vi "Remove and Rewire Objects_core.vi"(8 "error in (no error)":errorcluster, 10 "Clean Wires (T)":bool=TRUE, 11 "Items to Remove":refnum<vi>[](array[refnum])) -> (0 "error out":errorcluster, 3 "Any Items Removed?":bool)   [LabVIEW 2020]
uses:
  <vilib>/Utility/Data Type/Type Definitions/Data Type.ctl
  <vilib>/Utility/Data Type/NI_Data Type.lvlib
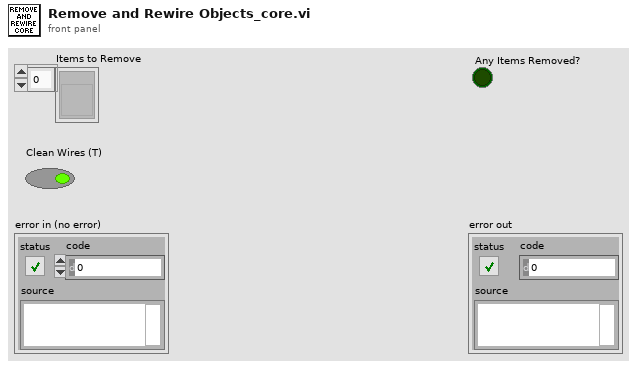
[diagram p1: front panel]
types:
  T1 = typedef "NI_Data Type.lvlib/Data Type.ctl" = enum8{"Invalid Type", "Void", "I8", "I16", "I32", "I64", "U8", "U16", "U32", "U64", "Single Float", "Double Float", "Extended Float", "Single Complex", "Double Complex", "Extended Complex", "Enum U8", "Enum U16", "Enum U32", "Enum U64", "Single Float With Unit", "Double Float With Unit", "Extended Float With Unit", "Single Complex with Unit", "Double Complex with Unit", "Extended Complex with Unit", "Boolean", "String", "Path", "Picture", "Tag", "Array", "Cluster", "Variant", "LV Variant", "Waveform", "Timestamp", "Digital Waveform", "Digital Data", "ExpressData", "Refnum", "External Data", "VI", "Poly VI", "LabVIEW Class Instance", "Fixed Point", "Set Collection", "Map Collection"}
  T2 = cluster{"Left":i32, "Top":i32, "Terminal":refnum<vi>}
  T3 = cluster{"Left":i32, "Top":i32, "Terminal":refnum<vi>}[]
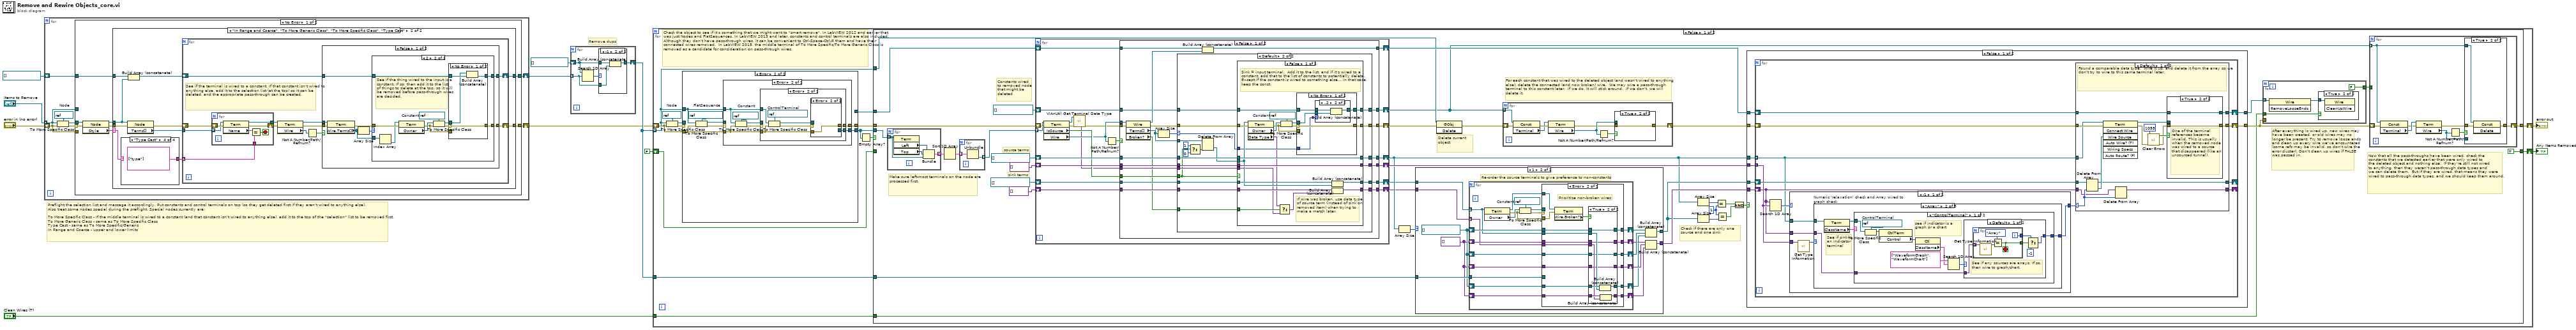
[diagram p0: block diagram]
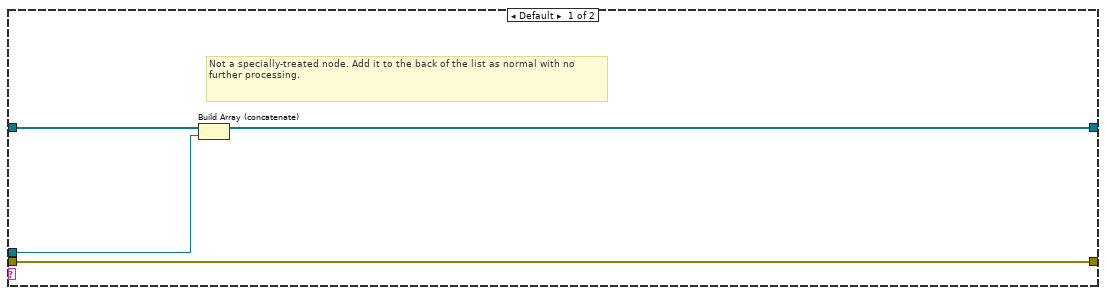
[diagram p3: hidden frame]
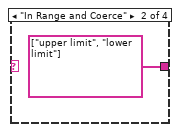
[diagram p5: hidden frame]
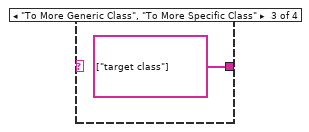
[diagram p6: hidden frame]
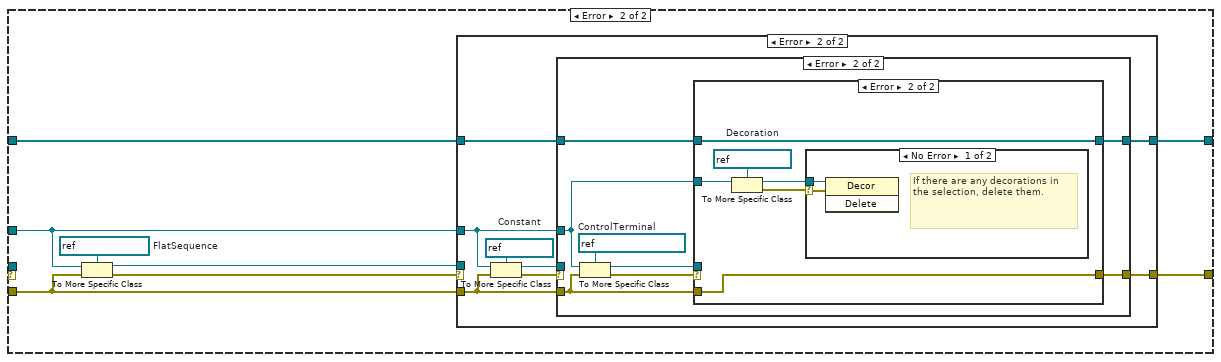
[diagram p10: hidden frame]
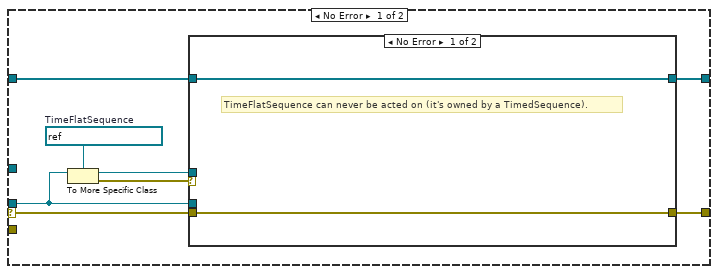
[diagram p11: hidden frame]
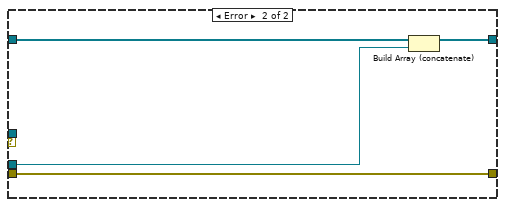
[diagram p12: hidden frame]
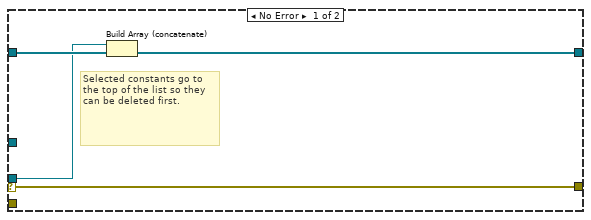
[diagram p13: hidden frame]
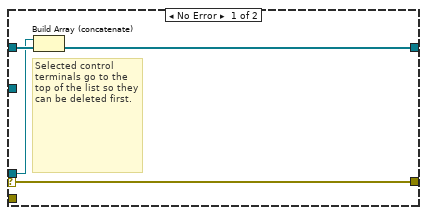
[diagram p14: hidden frame]
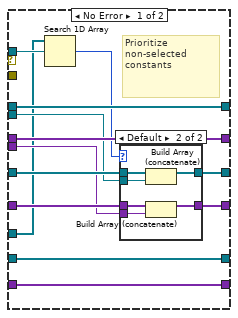
[diagram p17: hidden frame]
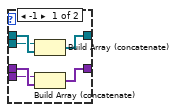
[diagram p18: hidden frame]
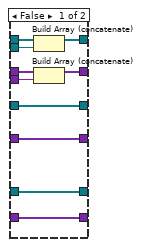
[diagram p19: hidden frame]
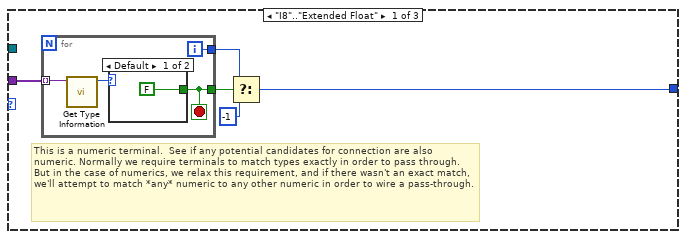
[diagram p20: hidden frame]
diagram:
  # "Preflight the selection list and massage it accordingly. Put constants and control terminals on top (so they get deleted first if they aren't wired to anything else).\nAlso treat some nodes special during the preflight. Special nodes currently are:\n\nTo More Specific Class - If the middle terminal is wired to a constant (and that constant isn't wired to anything else), add it to the top of the \"selection\" list to be removed first.\nTo More Generic Class - same as To More Specific Class\nType Cast - same as To More Specific/Generic\nIn Range and Coerce - upper and lower limits"
  # "Remove dups"
  n1 = for {
    tunnel: "Items to Remove" -> [w13] mode=indexing
    shift-right: [w14] -> w7
    shift-left: "error in (no error)" -> [w17]
    shift-right: [w15] -> w9
    shift-left: refnum<vi>[] [] ("SelList[]") -> [w16]
    w12 = refnum<vi> refnum  # Node
    n2 = To More Specific Class(target class=w12, reference=w13, error in=w17) -> (specific class reference=w19:refnum<vi>, error out=w18:errorcluster)
    n3 = case shown="No Error" w18 {
      selector: w18 -> [w27 _]
      tunnel: w19 -> [w26 _]
      tunnel: [w20 w98] -> w14
      tunnel: w13 -> [_ w96]
      tunnel: w17 -> [_ w97]
      tunnel: w16 -> [w22 w95]
      tunnel: [w21 w94] -> w15
      frame No Error {
        n4 = property class="Node"(reference=w26, error in=w27) -> (reference out=w23:refnum<vi>, error out=w24:errorcluster, "Style"=w25:string)
        n5 = case shown="\"In Range and Coerce\", \"To More Generic Class\", \"To More Specific Class\", \"Type Cast\"" w25 {
          selector: w25 -> [_ w32]
          tunnel: w24 -> [w29 w40]
          tunnel: w23 -> [w28 w39]
          tunnel: w22 -> [w31 w41]
          tunnel: [w30 w35] -> w21
          tunnel: [w29 w34] -> w20
          frame Default {
            # "Not a specially-treated node. Add it to the back of the list as normal with no further processing."
            n6 = Build Array (concatenate)(w31, w28) -> (w30:refnum<vi>[])
          }
          frame "In Range and Coerce", "To More Generic Class", "To More Specific Class", "Type Cast" {
            n7 = case shown="\"Type Cast\"" w32 {
              tunnel: [_ string[] ["upper limit", "lower limit"] string[] ["target class"] string[] ["type"]] -> w33
              frame Default {
              }
              frame "In Range and Coerce" {
              }
              frame "To More Generic Class", "To More Specific Class" {
              }
              frame "Type Cast" {
              }
            }
            n8 = property class="Node"(reference=w39, error in=w40) -> (error out=w38:errorcluster, "Terms[]"=w37:refnum<vi>[])  [unwired: 1 out]
            n9 = Build Array (concatenate)(w41, w39) -> (w36:refnum<vi>[])
            n10 = for {
              tunnel: w37 -> [w55]
              shift-right: [w51] -> w34
              shift-left: w38 -> [w56]
              shift-right: [w52] -> w35
              shift-left: w36 -> [w53]
              tunnel: w33 -> [w45] mode=indexing
              # "See if the terminal is wired to a constant. If that constant isn't wired to anything else, add it to the selection list (at the top) so it can be deleted, and the appropriate pass-through can be created."
              n11 = for {
                tunnel: w55 -> [w91] mode=indexing
                tunnel: [w89] -> w49
                shift-right: [w88] -> w54
                shift-left: w56 -> [w92]
                tunnel: w45 -> [w86]
                stop <- w87 stop-if-true
                n12 = property class="Term"(reference=w91, error in=w92) -> (reference out=w89:refnum<vi>, error out=w88:errorcluster, "Name"=w90:string)
                n13 = Equal?(x=w90, y=w86) -> (x = y?=w87:bool)
              }
              n14 = property class="Term"(reference=w49, error in=w54) -> (reference out=w48:refnum<vi>, error out=w50:errorcluster, "Wire"=w47:refnum<vi>)
              n15 = Not A Number/Path/Refnum?(number/path/refnum=w47) -> (NaN/Path/Refnum?=w46:bool)
              n16 = case shown="False" w46 {
                tunnel: w53 -> [w64 w85]
                tunnel: [w61 w85] -> w52
                tunnel: [w60 w84] -> w51
                tunnel: w50 -> [w58 w84]
                tunnel: w48 -> [w57 _]
                frame False {
                  n17 = property class="Term"(reference=w57, error in=w58) -> (error out=w63:errorcluster, "Wire.Terms[]"=w59:refnum<vi>[])  [unwired: 1 out]
                  n18 = Array Size(array=w59) -> (size(s)=w62:i32)
                  n19 = case shown="2" w62 {
                    tunnel: w64 -> [w66 w71]
                    tunnel: w63 -> [w65 w76]
                    tunnel: [w66 w70] -> w61
                    tunnel: [w65 w68] -> w60
                    tunnel: w59 -> [_ w77]
                    frame Default {
                      # "Any number of terminals on the upper/lower limit wires other than 2 means that whatever is wired to it, is also wired to something else. Don't try to delete that thing in this case."
                    }
                    frame 2 {
                      w73 = refnum<vi> refnum  # Constant
                      # "See if the thing wired to the input is a constant. If so, then add it to the list of things to delete at the top, so it will be removed before pass-through wires are decided."
                      n20 = Index Array(array=w77) -> (element=w75:refnum<vi>)  [unwired: 1 in]
                      n21 = property class="Term"(reference=w75, error in=w76) -> (error out=w69:errorcluster, "Owner"=w74:refnum<vi>)  [unwired: 1 out]
                      n22 = To More Specific Class(target class=w73, reference=w74, error in=w69) -> (specific class reference=w67:refnum<vi>, error out=w72:errorcluster)
                      n23 = case shown="No Error" w72 {
                        selector: w72 -> [w79 _]
                        tunnel: w71 -> [w81 w83]
                        tunnel: [w80 w83] -> w70
                        tunnel: w69 -> [_ w82]
                        tunnel: [w79 w82] -> w68
                        tunnel: w67 -> [w78 _]
                        frame No Error {
                          n24 = Build Array (concatenate)(w78, w81) -> (w80:refnum<vi>[])
                        }
                        frame Error {
                        }
                      }
                    }
                  }
                }
                frame True {
                  # "Terminal is not wired...no further work necessary"
                }
              }
            }
          }
        }
      }
      frame Error {
        w93 = refnum<vi> refnum  # FlatSequence
        n25 = To More Specific Class(target class=w93, reference=w96, error in=w97) -> (specific class reference=w99:refnum<vi>, error out=w100:errorcluster)
        n26 = case shown="Error" w100 {
          selector: w100 -> [w103 _]
          tunnel: w99 -> [w105 _]
          tunnel: [w102 w118] -> w98
          tunnel: w97 -> [_ w119]
          tunnel: w96 -> [_ w120]
          tunnel: w95 -> [w108 w117]
          tunnel: [w107 w116] -> w94
          frame No Error {
            w106 = refnum<vi> refnum  # TimeFlatSequence
            n27 = To More Specific Class(target class=w106, reference=w105) -> (specific class reference=w101:refnum<vi>, error out=w104:errorcluster)  [unwired: 1 in]
            n28 = case shown="No Error" w104 {
              tunnel: w108 -> [w109 w114]
              tunnel: [w109 w113] -> w107
              tunnel: w105 -> [_ w112]
              tunnel: w103 -> [w110 w111]
              tunnel: [w110 w111] -> w102
              tunnel: w101 -> [_ _]
              frame No Error {
                # "TimeFlatSequence can never be acted on (it's owned by a TimedSequence)."
              }
              frame Error {
                n29 = Build Array (concatenate)(w114, w112) -> (w113:refnum<vi>[])
              }
            }
          }
          frame Error {
            w115 = refnum<vi> refnum  # Constant
            n30 = To More Specific Class(target class=w115, reference=w120, error in=w119) -> (specific class reference=w121:refnum<vi>, error out=w122:errorcluster)
            n31 = case shown="Error" w122 {
              selector: w122 -> [w126 _]
              tunnel: w121 -> [w123 _]
              tunnel: w120 -> [_ w127]
              tunnel: w119 -> [_ w132]
              tunnel: [w126 w131] -> w118
              tunnel: w117 -> [w125 w130]
              tunnel: [w124 w129] -> w116
              frame No Error {
                # "Selected constants go to the top of the list so they can be deleted first."
                n32 = Build Array (concatenate)(w123, w125) -> (w124:refnum<vi>[])
              }
              frame Error {
                w128 = refnum<vi> refnum  # ControlTerminal
                n33 = To More Specific Class(target class=w128, reference=w127, error in=w132) -> (specific class reference=w133:refnum<vi>, error out=w134:errorcluster)
                n34 = case shown="Error" w134 {
                  selector: w134 -> [w138 _]
                  tunnel: w133 -> [w135 _]
                  tunnel: w132 -> [_ w144]
                  tunnel: [w138 w144] -> w131
                  tunnel: w130 -> [w137 w143]
                  tunnel: [w136 w143] -> w129
                  tunnel: w127 -> [_ w142]
                  frame No Error {
                    # "Selected control terminals go to the top of the list so they can be deleted first."
                    n35 = Build Array (concatenate)(w135, w137) -> (w136:refnum<vi>[])
                  }
                  frame Error {
                    w141 = refnum<vi> refnum  # Decoration
                    n36 = To More Specific Class(target class=w141, reference=w142) -> (specific class reference=w139:refnum<vi>, error out=w140:errorcluster)  [unwired: 1 in]
                    n37 = case shown="No Error" w140 {
                      selector: w140 -> [w145 _]
                      tunnel: w139 -> [w146 _]
                      frame No Error {
                        # "If there are any decorations in the selection, delete them."
                        n38 = invoke class="Decor" method="Delete"(reference=w146, error in=w145) -> ()  [unwired: 1 in, 3 out]
                      }
                      frame Error {
                      }
                    }
                  }
                }
              }
            }
          }
        }
      }
    }
  }
  n39 = for {
    tunnel: w9 -> [w147] mode=indexing
    shift-right: [w148] -> w11
    shift-left: refnum<vi>[] [] ("SelList[]") -> [w149]
    n40 = Search 1D Array(1D array=w149, element=w147) -> (index of element=w150:i32)  [unwired: 1 in]
    n41 = case shown="-1" w150 {
      tunnel: w149 -> [w151 w154]
      tunnel: [w151 w153] -> w148
      tunnel: w147 -> [_ w152]
      frame Default {
      }
      frame -1 {
        n42 = Build Array (concatenate)(w154, w152) -> (w153:refnum<vi>[])
      }
    }
  }
  n43 = for {
    tunnel: w11 -> [w162] mode=indexing
    shift-right: [w161] -> w3
    shift-left: FALSE -> [w156]
    shift-right: [w160] -> w4
    shift-left: w7 -> [w166]
    tunnel: w11 -> [w159]
    tunnel: "Clean Wires (T)" -> [w155]
    w158 = refnum<vi> refnum  # Node
    # "Check the object to see if it's something that we might want to \"smart remove\". In LabVIEW 2012 and earlier that was just Nodes and FlatSequences. In LabVIEW 2013 and later, constants and control terminals are also included. Although they don't have pass-through wires, it can be convenient to Ctrl-Space-Ctrl-R them and have their connected wires removed.  In LabVIEW 2015, the middle terminal of To More Specific/To More Generic Class is removed as a candidate for consideration on pass-through wires."
    n44 = To More Specific Class(target class=w158, reference=w162, error in=w166) -> (specific class reference=w167:refnum<vi>, error out=w168:errorcluster)
    n45 = case shown="Error" w168 {
      selector: w168 -> [w573 _]
      tunnel: w167 -> [w572 _]
      tunnel: [w569 w599] -> w163
      tunnel: [w567 w601] -> w164
      tunnel: w162 -> [_ w598]
      tunnel: w166 -> [_ w600]
      tunnel: [w568 _] -> w157
      frame No Error {
        # "Ignored terminals:\nTo More Specific - middle terminal\nTo More Generic - middle terminal\nType Cast - middle terminal\nIn Range and Coerce - upper and lower limit terminals"
        n46 = property class="Node"(reference=w572, error in=w573) -> (error out=w567:errorcluster, "Terms[]"=w570:refnum<vi>[], "Style"=w571:string)  [unwired: 1 out]
        n47 = case "Don't look at certain terminals on certain nodes" shown="\"In Range and Coerce\"" w571 {
          tunnel: w570 -> [w579 w585 w595 w596]
          tunnel: [w577 w583 w589 w596] -> w569
          tunnel: [w574 w580 w591 _] -> w568
          frame "To More Generic Class", "Type Cast" {
            n48 = Delete From Array(array=w579, index=1) -> (deleted portion=w575:refnum<vi>, array with subset deleted=w577:refnum<vi>[])  [unwired: 1 in]
            n49 = property class="Term"(reference=w575) -> ("Wire"=w576:refnum<vi>)  [unwired: 1 in, 2 out]
            n50 = Build Array(w576) -> (w574:refnum<vi>[])
          }
          frame "To More Specific Class" {
            n51 = Delete From Array(array=w585, index=2) -> (deleted portion=w581:refnum<vi>, array with subset deleted=w583:refnum<vi>[])  [unwired: 1 in]
            n52 = property class="Term"(reference=w581) -> ("Wire"=w582:refnum<vi>)  [unwired: 1 in, 2 out]
            n53 = Build Array(w582) -> (w580:refnum<vi>[])
          }
          frame "In Range and Coerce" {
            n54 = Delete From Array(array=w595, index=4) -> (deleted portion=w592:refnum<vi>, array with subset deleted=w590:refnum<vi>[])  [unwired: 1 in]
            n55 = Delete From Array(array=w590, index=2) -> (deleted portion=w587:refnum<vi>, array with subset deleted=w589:refnum<vi>[])  [unwired: 1 in]
            n56 = property class="Term"(reference=w587) -> ("Wire"=w586:refnum<vi>)  [unwired: 1 in, 2 out]
            n57 = property class="Term"(reference=w592) -> ("Wire"=w593:refnum<vi>)  [unwired: 1 in, 2 out]
            n58 = Build Array(w586, w593) -> (w591:refnum<vi>[])
          }
          frame Default {
          }
        }
      }
      frame Error {
        w597 = refnum<vi> refnum  # FlatSequence
        n59 = To More Specific Class(target class=w597, reference=w598, error in=w600) -> (specific class reference=w602:refnum<vi>, error out=w603:errorcluster)
        n60 = case shown="Error" w603 {
          selector: w603 -> [w607 _]
          tunnel: w602 -> [w606 _]
          tunnel: [w605 w609] -> w601
          tunnel: w600 -> [_ w611]
          tunnel: [w604 w610] -> w599
          tunnel: w598 -> [_ w612]
          frame No Error {
            n61 = property class="FlatSeq"(reference=w606, error in=w607) -> (error out=w605:errorcluster, "Terms[]"=w604:refnum<vi>[])  [unwired: 1 out]
          }
          frame Error {
            w608 = refnum<vi> refnum  # Constant
            n62 = To More Specific Class(target class=w608, reference=w612, error in=w611) -> (specific class reference=w613:refnum<vi>, error out=w614:errorcluster)
            n63 = case shown="Error" w614 {
              selector: w614 -> [w618 _]
              tunnel: w613 -> [w619 _]
              tunnel: w612 -> [_ w626]
              tunnel: w611 -> [_ w623]
              tunnel: [w616 w621] -> w610
              tunnel: [w615 w622] -> w609
              frame No Error {
                n64 = property class="Const"(reference=w619, error in=w618) -> (error out=w615:errorcluster, "Terminal"=w617:refnum<vi>)  [unwired: 1 out]
                n65 = Build Array(w617) -> (w616:refnum<vi>[])
              }
              frame Error {
                w620 = refnum<vi> refnum  # ControlTerminal
                n66 = To More Specific Class(target class=w620, reference=w626, error in=w623) -> (specific class reference=w624:refnum<vi>, error out=w625:errorcluster)
                n67 = case shown="Error" w625 {
                  selector: w625 -> [w629 _]
                  tunnel: w624 -> [w628 _]
                  tunnel: w623 -> [_ w630]
                  tunnel: [w629 w630] -> w622
                  tunnel: [w627 _] -> w621
                  frame No Error {
                    n68 = Build Array(w628) -> (w627:refnum<vi>[])
                  }
                  frame Error {
                  }
                }
              }
            }
          }
        }
      }
    }
    n69 = Empty Array?(array=w163) -> (empty?=w165:bool)
    n70 = case shown="False" w165 {
      tunnel: w164 -> [w205 w566]
      tunnel: [w191 w566] -> w160
      tunnel: w156 -> [_ w565]
      tunnel: w163 -> [w173 _]
      tunnel: w162 -> [w195 _]
      tunnel: [TRUE w565] -> w161
      tunnel: w159 -> [w178 _]
      tunnel: w157 -> [w171 _]
      tunnel: w155 -> [w169 _]
      frame False {
        w187 = 1 ("y")
        # "Make sure left-most terminals on the node are processed first."
        # "Check if there are only one source and one sink"
        # "Now that all the pass-throughs have been wired, check the\nconstants that we detected earlier that were only wired to\nthe deleted object and nothing else.  If they're still not wired\nto anything, then they weren't pass-through data types and\nwe can delete them.  But if they are wired, that means they were\nwired to pass-through data types, and we should keep them around."
        # "For each constant that was wired to the deleted object (and wasn't wired to anything\nelse), delete the connected (and now broken) wire.  We may wire a pass-through\nterminal to this constant later.  If we do, it will stick around.  If we don't, we will\ndelete it."
        # "Constants wired\nto removed node\nthat might be\ndeleted"
        # "After everything is wired up, new wires may have been created, or old wires may no longer be present. Try to remove loose ends and clean up every wire we've encountered (some refs may be invalid, so don't wire the error cluster). Don't clean up wires if FALSE was passed in."
        # "Delete current object"
        # "sink terms"
        # "source terms"
        n71 = for {
          tunnel: w173 -> [w209] mode=indexing
          tunnel: [w210] -> w175 mode=indexing
          n72 = property class="Term"(reference=w209) -> ("Left"=w211:i32, "Top"=w208:i32)  [unwired: 1 in, 2 out]
          n73 = Bundle("Left"=w211, "Top"=w208, "Terminal"=w209) -> (w210:T2)  [unwired: 1 in]
        }
        n74 = Sort 1D Array(array=w175) -> (sorted array=w174:T3)
        n75 = for {
          tunnel: w174 -> [w207] mode=indexing
          tunnel: [w206] -> w172 mode=indexing
          n76 = Unbundle(w207) -> ("Terminal"=w206:refnum<vi>)  [unwired: 2 out]
        }
        n77 = for {
          shift-right: [w454] -> w199
          shift-left: w205 -> [w465]
          tunnel: w172 -> [w464] mode=indexing
          shift-right: [w457] -> w180
          shift-left: refnum<vi>[] [] -> [w463]
          shift-right: [w456] -> w183
          shift-left: variant[] [] -> [w462]
          shift-right: [w459] -> w177
          shift-left: refnum<vi>[] [] -> [w461]
          shift-right: [w458] -> w176
          shift-left: variant[] [] -> [w460]
          shift-right: [w450] -> w198
          shift-left: w171 -> [w451]
          shift-right: [w448] -> w190
          shift-left: refnum<vi>[] [] -> [w449]
          n78 = property class="Term"(reference=w464, error in=w465) -> (reference out=w446:refnum<vi>, error out=w447:errorcluster, "IsSource"=w455:bool, "Wire"=w453:refnum<vi>)
          n79 = call <vilib>:"VIAnUtil Get Terminal Data Type.vi"("error in (no error)"=w447, "Terminal in"=w446) -> ("error out"=w444:errorcluster, "Type Variant"=w445:variant)  [unwired: 6 in, 2 out]
          n80 = Not A Number/Path/Refnum?(number/path/refnum=w453) -> (NaN/Path/Refnum?=w452:bool)
          n81 = case shown="False" w452 {
            tunnel: w463 -> [w487 w562]
            tunnel: w462 -> [w486 w561]
            tunnel: w461 -> [w485 w560]
            tunnel: w460 -> [w484 w559]
            tunnel: w445 -> [w483 _]
            tunnel: [w482 w560] -> w459
            tunnel: [w481 w559] -> w458
            tunnel: [w480 w562] -> w457
            tunnel: [w479 w561] -> w456
            tunnel: w444 -> [w478 w563]
            tunnel: w455 -> [w476 _]
            tunnel: [w470 w563] -> w454
            tunnel: w453 -> [w477 _]
            tunnel: w451 -> [w475 w564]
            tunnel: [w474 w564] -> w450
            tunnel: w449 -> [w471 w558]
            tunnel: [w469 w558] -> w448
            frame False {
              n82 = property class="Wire"(reference=w477, error in=w478) -> (reference out=w473:refnum<vi>, error out=w472:errorcluster, "Terms[]"=w468:refnum<vi>[], "Broken?"=w466:bool)
              n83 = Array Size(array=w468) -> (size(s)=w467:i32)
              n84 = case shown="Default" w467 {
                selector: w467 -> [_ w496]
                tunnel: w487 -> [w491 w515]
                tunnel: w486 -> [w492 w514]
                tunnel: w485 -> [w493 w513]
                tunnel: w484 -> [w494 w512]
                tunnel: w483 -> [_ w511]
                tunnel: [w493 w510] -> w482
                tunnel: [w494 w509] -> w481
                tunnel: [w491 w508] -> w480
                tunnel: [w492 w507] -> w479
                tunnel: w476 -> [_ w502]
                tunnel: w472 -> [w488 w501]
                tunnel: w471 -> [w490 w500]
                tunnel: [w488 w499] -> w470
                tunnel: [w490 w498] -> w469
                tunnel: w468 -> [w489 w497]
                tunnel: w466 -> [_ w495]
                frame 1 {
                  # "If the wire only has one terminal, then it is a broken wire, with either no source\nor no sink.  Don't try to get data type information on this wire, as it will end up\nbeing removed by the \"Remove Loose Ends\" call later (note that we're still adding\nthe wire to the wires array above)."
                  n85 = Close Reference(reference=w489) -> ()  [unwired: 1 in, 1 out]
                }
                frame Default {
                  n86 = Select(t=1, s=w502, f=0) -> (s? t:f=w504:i32)
                  n87 = Delete From Array(array=w497, index=w504) -> (deleted portion=w503:refnum<vi>)  [unwired: 1 in, 1 out]
                  n88 = case shown="False" w502 {
                    tunnel: w515 -> [w534 w555]
                    tunnel: w514 -> [w533 w553]
                    tunnel: w513 -> [w536 w557]
                    tunnel: w512 -> [w535 w556]
                    tunnel: w511 -> [w519 w550]
                    tunnel: w503 -> [w522 w554]
                    tunnel: [w532 w557] -> w510
                    tunnel: [w531 w556] -> w509
                    tunnel: [w534 w552] -> w508
                    tunnel: [w533 w551] -> w507
                    tunnel: w501 -> [w530 w549]
                    tunnel: w500 -> [w524 w548]
                    tunnel: [w525 w549] -> w499
                    tunnel: [w523 w548] -> w498
                    tunnel: w496 -> [w521 _]
                    tunnel: w495 -> [w520 _]
                    frame False {
                      w516 = refnum<vi> refnum  # Constant
                      # "If wire was broken, use data type of source term (instead of sink on removed item) when trying to make a match later."
                      # "Sink = input terminal.  Add it to the list, and if it's wired to a constant, add that to the list of constants to potentially delete.  Except if the constant is wired to something else... in that case, keep the const."
                      n89 = property class="Term"(reference=w522, error in=w530) -> (error out=w526:errorcluster, "Owner"=w529:refnum<vi>, "Data Type"=w517:variant)  [unwired: 1 out]
                      n90 = Select(t=w517, s=w520, f=w519) -> (s? t:f=w518:variant)
                      n91 = To More Specific Class(target class=w516, reference=w529, error in=w526) -> (specific class reference=w527:refnum<vi>, error out=w528:errorcluster)
                      n92 = case shown="No Error" w528 {
                        selector: w528 -> [w539 _]
                        tunnel: w527 -> [w538 _]
                        tunnel: w526 -> [_ w547]
                        tunnel: [w539 w547] -> w525
                        tunnel: [w540 w546] -> w523
                        tunnel: w524 -> [w541 w546]
                        tunnel: w521 -> [w537 _]
                        frame No Error {
                          n93 = case shown="..2" w537 {
                            tunnel: w541 -> [w542 w545]
                            tunnel: [w542 w544] -> w540
                            tunnel: w538 -> [_ w543]
                            frame 3.. {
                            }
                            frame ..2 {
                              n94 = Build Array (concatenate)(w545, w543) -> (w544:refnum<vi>[])
                            }
                          }
                        }
                        frame Error {
                        }
                      }
                      n95 = Build Array (concatenate)(w536, w522) -> (w532:refnum<vi>[])
                      n96 = Build Array (concatenate)(w535, w518) -> (w531:variant[])
                    }
                    frame True {
                      # "Source = output terminal.  Add it to the list."
                      n97 = Build Array (concatenate)(w555, w554) -> (w552:refnum<vi>[])
                      n98 = Build Array (concatenate)(w553, w550) -> (w551:variant[])
                    }
                  }
                }
              }
              n99 = Build Array (concatenate)(w475, w473) -> (w474:refnum<vi>[])
            }
            frame True {
              # "This terminal isn't wired to anything.  Ignore it."
            }
          }
        }
        n100 = Array Size(array=w180) -> (size(s)=w179:i32)
        n101 = case shown="1" w179 {
          tunnel: w177 -> [w213 w226]
          tunnel: w176 -> [w212 w225]
          tunnel: [w212 w224] -> w182
          tunnel: [w213 w223] -> w181
          tunnel: w178 -> [_ w218]
          frame Default {
          }
          frame 1 {
            w216 = variant[] []
            w217 = refnum<vi>[] []
            # "Re-order the source terminals to give preference to non-constants"
            n102 = for {
              tunnel: w226 -> [w238] mode=indexing
              tunnel: w225 -> [w239] mode=indexing
              shift-right: [w241] -> w222
              shift-left: w217 -> [w243]
              shift-right: [w240] -> w220
              shift-left: w216 -> [w242]
              shift-right: [w236] -> w221
              shift-left: w217 -> [w237]
              shift-right: [w234] -> w219
              shift-left: w216 -> [w235]
              tunnel: w218 -> [w233]
              shift-right: [w228] -> w215
              shift-left: w217 -> [w230]
              shift-right: [w227] -> w214
              shift-left: w216 -> [w229]
              w246 = refnum<vi> refnum  # Constant
              n103 = property class="Term"(reference=w238) -> (reference out=w232:refnum<vi>, error out=w231:errorcluster, "Owner"=w247:refnum<vi>)  [unwired: 1 in]
              n104 = To More Specific Class(target class=w246, reference=w247, error in=w231) -> (specific class reference=w244:refnum<vi>, error out=w245:errorcluster)
              n105 = case shown="Error" w245 {
                tunnel: w244 -> [w252 _]
                tunnel: w243 -> [w260 w289]
                tunnel: w242 -> [w259 w288]
                tunnel: [w260 w287] -> w241
                tunnel: [w259 w286] -> w240
                tunnel: w239 -> [w253 w285]
                tunnel: w238 -> [w257 w284]
                tunnel: [w256 w275] -> w236
                tunnel: w237 -> [w258 w276]
                tunnel: w235 -> [w255 w274]
                tunnel: [w254 w273] -> w234
                tunnel: w233 -> [w251 _]
                tunnel: w232 -> [_ w282]
                tunnel: w231 -> [_ w283]
                tunnel: w230 -> [w249 w279]
                tunnel: w229 -> [w248 w277]
                tunnel: [w249 w280] -> w228
                tunnel: [w248 w278] -> w227
                frame No Error {
                  # "Prioritize non-selected constants"
                  n106 = Search 1D Array(1D array=w251, element=w252) -> (index of element=w250:i32)  [unwired: 1 in]
                  n107 = case shown="Default" w250 {
                    tunnel: w258 -> [w266 w272]
                    tunnel: w257 -> [w265 w271]
                    tunnel: [w264 w270] -> w256
                    tunnel: w255 -> [w263 w269]
                    tunnel: [w262 w268] -> w254
                    tunnel: w253 -> [w261 w267]
                    frame -1 {
                      n108 = Build Array (concatenate)(w265, w266) -> (w264:refnum<vi>[])
                      n109 = Build Array (concatenate)(w261, w263) -> (w262:variant[])
                    }
                    frame Default {
                      n110 = Build Array (concatenate)(w272, w271) -> (w270:refnum<vi>[])
                      n111 = Build Array (concatenate)(w269, w267) -> (w268:variant[])
                    }
                  }
                }
                frame Error {
                  # "Prioritize non-broken wires"
                  n112 = property class="Term"(reference=w282, error in=w283) -> ("Wire.Broken?"=w281:bool)  [unwired: 2 out]
                  n113 = case shown="True" w281 {
                    tunnel: w289 -> [w299 w303]
                    tunnel: w288 -> [w296 w302]
                    tunnel: [w298 w303] -> w287
                    tunnel: [w295 w302] -> w286
                    tunnel: w285 -> [w294 w304]
                    tunnel: w284 -> [w297 w307]
                    tunnel: [w293 w309] -> w280
                    tunnel: w279 -> [w293 w308]
                    tunnel: [w292 w306] -> w278
                    tunnel: w277 -> [w292 w305]
                    tunnel: w276 -> [w291 w301]
                    tunnel: [w291 w301] -> w275
                    tunnel: w274 -> [w290 w300]
                    tunnel: [w290 w300] -> w273
                    frame False {
                      n114 = Build Array (concatenate)(w299, w297) -> (w298:refnum<vi>[])
                      n115 = Build Array (concatenate)(w296, w294) -> (w295:variant[])
                    }
                    frame True {
                      n116 = Build Array (concatenate)(w308, w307) -> (w309:refnum<vi>[])
                      n117 = Build Array (concatenate)(w305, w304) -> (w306:variant[])
                    }
                  }
                }
              }
            }
            n118 = Build Array (concatenate)(w222, w221, w215) -> (w223:refnum<vi>[])
            n119 = Build Array (concatenate)(w220, w219, w214) -> (w224:variant[])
          }
        }
        n120 = invoke class="GObj" method="Delete"(reference=w195, error in=w199) -> (error out=w194:errorcluster)  [unwired: 1 in, 2 out]
        n121 = for {
          tunnel: w190 -> [w433] mode=indexing
          shift-right: [w430] -> w193
          shift-left: w194 -> [w434]
          n122 = property class="Const"(reference=w433, error in=w434) -> (error out=w432:errorcluster, "Terminal"=w431:refnum<vi>)  [unwired: 1 out]
          n123 = property class="Term"(reference=w431, error in=w432) -> (error out=w427:errorcluster, "Wire"=w429:refnum<vi>)  [unwired: 1 out]
          n124 = Not A Number/Path/Refnum?(number/path/refnum=w429) -> (NaN/Path/Refnum?=w428:bool)
          n125 = case shown="True" w428 {
            tunnel: w427 -> [w437 w438]
            tunnel: [w436 w438] -> w430
            tunnel: w429 -> [w435 _]
            frame False {
              n126 = invoke class="Wire" method="Delete"(reference=w435, error in=w437) -> (error out=w436:errorcluster)  [unwired: 1 in, 2 out]
            }
            frame True {
            }
          }
        }
        n127 = Array Size(array=w180) -> (size(s)=w189:i32)
        n128 = Array Size(array=w181) -> (size(s)=w188:i32)
        n129 = Equal?(x=w189, y=w187) -> (x = y?=w186:bool)
        n130 = Equal?(x=w187, y=w188) -> (x = y?=w185:bool)
        n131 = And(x=w186, y=w185) -> (x .and. y?=w184:bool)
        n132 = case shown="False" w184 {
          tunnel: w183 -> [w317 _]
          tunnel: w182 -> [w316 _]
          tunnel: w198 -> [w315 w407]
          tunnel: [w314 w405] -> w197
          tunnel: w193 -> [w313 w412]
          tunnel: [w312 w402] -> w192
          tunnel: w180 -> [w311 w414]
          tunnel: w181 -> [w310 w413]
          frame False {
            n133 = for {
              shift-right: [w325] -> w312
              shift-left: w313 -> [w327]
              tunnel: w311 -> [w318] mode=indexing
              tunnel: w317 -> [w320] mode=indexing
              shift-right: [w328] -> w314
              shift-left: w315 -> [w329]
              shift-right: [w324] -> _
              shift-left: w310 -> [w326]
              shift-right: [w323] -> _
              shift-left: w316 -> [w319]
              n134 = Search 1D Array(1D array=w319, element=w320) -> (index of element=w322:i32)  [unwired: 1 in]
              n135 = case shown="-1" w322 {
                selector: w322 -> [_ w373]
                tunnel: [w331 w373] -> w321
                tunnel: w320 -> [w334 _]
                tunnel: w319 -> [w332 _]
                tunnel: w318 -> [w330 _]
                frame -1 {
                  n136 = call <vilib>:"Get Type Information.vi"("variant"=w334) -> ("type"=w333:T1)  [unwired: 6 in, 4 out]
                  n137 = case "Numeric 'relaxation' check and Array wired to graph check" shown="\"Array\"" w333 {
                    tunnel: w332 -> [w339 w346 _]
                    tunnel: [w335 w349 -1] -> w331
                    tunnel: w330 -> [_ w350 _]
                    frame "I8".."Extended Float" {
                      # "This is a numeric terminal.  See if any potential candidates for connection are also numeric. Normally we require terminals to match types exactly in order to pass through.  But in the case of numerics, we relax this requirement, and if there wasn't an exact match, we'll attempt to match *any* numeric to any other numeric in order to wire a pass-through."
                      n138 = for {
                        tunnel: w339 -> [w343] mode=indexing
                        tunnel: [w341] -> w338
                        tunnel: [w340] -> w337
                        i -> [w340]
                        stop <- w341 stop-if-true
                        n139 = call <vilib>:"Get Type Information.vi"("variant"=w343) -> ("type"=w342:T1)  [unwired: 6 in, 4 out]
                        n140 = case shown="Default" w342 {
                          tunnel: [FALSE TRUE] -> w341
                          frame Default {
                          }
                          frame "I8".."Extended Float" {
                          }
                        }
                      }
                      n141 = Select(t=w337, s=w338, f=-1) -> (s? t:f=w335:i32)
                    }
                    frame "Array" {
                      # "See if sink is an indicator terminal"
                      n142 = property class="Term"(reference=w350) -> (reference out=w347:refnum<vi>, "ClassName"=w348:string)  [unwired: 1 in, 1 out]
                      n143 = case shown="\"ControlTerminal\"" w348 {
                        tunnel: [w352 -1] -> w349
                        tunnel: w347 -> [w359 _]
                        tunnel: w346 -> [w351 _]
                        frame "ControlTerminal" {
                          w358 = refnum<vi> refnum  # ControlTerminal
                          # "see if indicator is a graph or a chart"
                          n144 = To More Specific Class(target class=w358, reference=w359) -> (specific class reference=w357:refnum<vi>)  [unwired: 1 in, 1 out]
                          n145 = property class="CtrlTerm"(reference=w357) -> ("Control"=w356:refnum<vi>)  [unwired: 1 in, 2 out]
                          n146 = property class="Ctl"(reference=w356) -> ("ClassName"=w354:string)  [unwired: 1 in, 2 out]
                          n147 = Search 1D Array(1D array=string[] ["WaveformGraph", "WaveformChart"], element=w354) -> (index of element=w353:i32)  [unwired: 1 in]
                          n148 = case shown="Default" w353 {
                            tunnel: [w361 -1] -> w352
                            tunnel: w351 -> [w364 _]
                            frame Default {
                              # "See if any sources are arrays. If so, then wire to graph/chart."
                              n149 = for {
                                tunnel: w364 -> [w369] mode=indexing
                                tunnel: [w366] -> w363
                                tunnel: [w365] -> w362
                                i -> [w365]
                                stop <- w366 stop-if-true
                                n150 = call <vilib>:"Get Type Information.vi"("variant"=w369) -> ("type"=w368:T1)  [unwired: 6 in, 4 out]
                                n151 = Equal?(x=Data_Type."Array", y=w368) -> (x = y?=w366:bool)
                              }
                              n152 = Select(t=w362, s=w363, f=-1) -> (s? t:f=w361:i32)
                            }
                            frame -1 {
                              # "Wired terminal is not a graph or chart"
                            }
                          }
                        }
                        frame Default {
                          # "The terminal is not an indicator terminal. This is not a graph/chart sink."
                        }
                      }
                    }
                    frame Default {
                      # "Not a numeric type or an array that might be wired to a chart/graph.\nDon't try to 'relax' it."
                    }
                  }
                }
                frame Default {
                  # "Exact match was found.  Use it."
                }
              }
              n153 = case shown="Default" w321 {
                selector: w321 -> [w379 _]
                tunnel: w329 -> [w384 w401]
                tunnel: [w383 w401] -> w328
                tunnel: w327 -> [w388 w400]
                tunnel: w318 -> [w387 _]
                tunnel: w326 -> [w389 w399]
                tunnel: [w382 w400] -> w325
                tunnel: [w381 w399] -> w324
                tunnel: w319 -> [w378 w398]
                tunnel: [w380 w398] -> w323
                frame Default {
                  # "Found a comparable data type.  Wire it up, and delete it from the array so we don't try to wire to this same terminal later."
                  n154 = Delete From Array(array=w389, index=w379) -> (deleted portion=w386:refnum<vi>, array with subset deleted=w381:refnum<vi>[])  [unwired: 1 in]
                  n155 = invoke class="Term" method="Connect Wire"(reference=w387, error in=w388, "Wire Source"=w386) -> (reference out=w385:refnum<vi>, error out=w375:errorcluster)  [unwired: 4 in, 5 out]
                  n156 = Delete From Array(array=w378, index=w379) -> (array with subset deleted=w380:variant[])  [unwired: 1 in, 1 out]
                  n157 = call <vilib>:"Clear Errors.vi"("error in (no error)"=w375, "specific error code to clear (0: all)"=1055) -> ("error out"=w374:errorcluster, "specific error cleared?"=w376:bool)  [unwired: 4 in]
                  n158 = case shown="True" w376 {
                    tunnel: w385 -> [w395 _]
                    tunnel: w384 -> [w394 w397]
                    tunnel: [w392 w397] -> w383
                    tunnel: [w391 w396] -> w382
                    tunnel: w374 -> [w390 w396]
                    frame False {
                      n159 = property class="Term"(reference=w395, error in=w390) -> (error out=w391:errorcluster, "Wire"=w393:refnum<vi>)  [unwired: 1 out]
                      n160 = Build Array (concatenate)(w394, w393) -> (w392:refnum<vi>[])
                    }
                    frame True {
                      # "One of the terminal references became invalid. This is usually when the removed node was wired to a source that disappeared (like an unsourced tunnel)."
                    }
                  }
                }
                frame -1 {
                  # "No comparable data type found for this item. Don't try to wire it up."
                }
              }
            }
          }
          frame True {
            # "Clear error 1055 for the case where one of the terminals is no longer valid. This is usually when a terminal that was sourced by a wire connected to the object completely disappears, like a tunnel on a structure that isn't wired on the inside."
            # "If there is only one source and one sink, go ahead and wire them up, don't bother doing the data type check. This solves the problem where there was originally a broken wire because data types didn't match, and the mismatch caused us to not try to rewire the source and sink."
            n161 = Index Array(array=w414) -> (element=w411:refnum<vi>)  [unwired: 1 in]
            n162 = Index Array(array=w413) -> (element=w410:refnum<vi>)  [unwired: 1 in]
            n163 = invoke class="Term" method="Connect Wire"(reference=w411, error in=w412, "Wire Source"=w410) -> (reference out=w409:refnum<vi>, error out=w408:errorcluster)  [unwired: 4 in, 5 out]
            n164 = property class="Term"(reference=w409, error in=w408) -> (error out=w403:errorcluster, "Wire"=w406:refnum<vi>)  [unwired: 1 out]
            n165 = Build Array (concatenate)(w407, w406) -> (w405:refnum<vi>[])
            n166 = call <vilib>:"Clear Errors.vi"("error in (no error)"=w403, "specific error code to clear (0: all)"=1055) -> ("error out"=w402:errorcluster)  [unwired: 4 in, 1 out]
          }
        }
        n167 = for {
          tunnel: w197 -> [w442] mode=indexing
          tunnel: w192 -> [_]
          tunnel: [FALSE] -> w170
          tunnel: w169 -> [w439]
          n168 = invoke class="Wire" method="RemoveLooseEnds"(reference=w442) -> (reference out=w441:refnum<vi>)  [unwired: 2 in, 2 out]
          n169 = case shown="True" w439 {
            tunnel: w441 -> [_ w443]
            frame False {
            }
            frame True {
              n170 = invoke class="Wire" method="CleanUpWire"(reference=w443) -> ()  [unwired: 2 in, 3 out]
            }
          }
        }
        n171 = for {
          shift-right: [w416] -> w191
          shift-left: w192 -> [w420]
          tunnel: w190 -> [w418] mode=indexing
          tunnel: w170 -> [_]
          n172 = property class="Const"(reference=w418, error in=w420) -> (error out=w421:errorcluster, "Terminal"=w422:refnum<vi>)  [unwired: 1 out]
          n173 = property class="Term"(reference=w422, error in=w421) -> (error out=w415:errorcluster, "Wire"=w417:refnum<vi>)  [unwired: 1 out]
          n174 = Not A Number/Path/Refnum?(number/path/refnum=w417) -> (NaN/Path/Refnum?=w419:bool)
          n175 = case shown="True" w419 {
            tunnel: w415 -> [w423 w425]
            tunnel: w418 -> [_ w424]
            tunnel: w417 -> [_ _]
            tunnel: [w423 w426] -> w416
            frame False {
            }
            frame True {
              n176 = invoke class="Const" method="Delete"(reference=w424, error in=w425) -> (error out=w426:errorcluster)  [unwired: 1 in, 2 out]
            }
          }
        }
      }
      frame True {
        # "Invalid object class, ignore this item."
      }
    }
  }
  "error out" <- w4
  "Any Items Removed?" <- w3
